vi "Screen.vi"() -> (1 "Screen":bool[][](array[boolean]))   [LabVIEW 2012]
panel:
  # "This screen is 100 x 150"
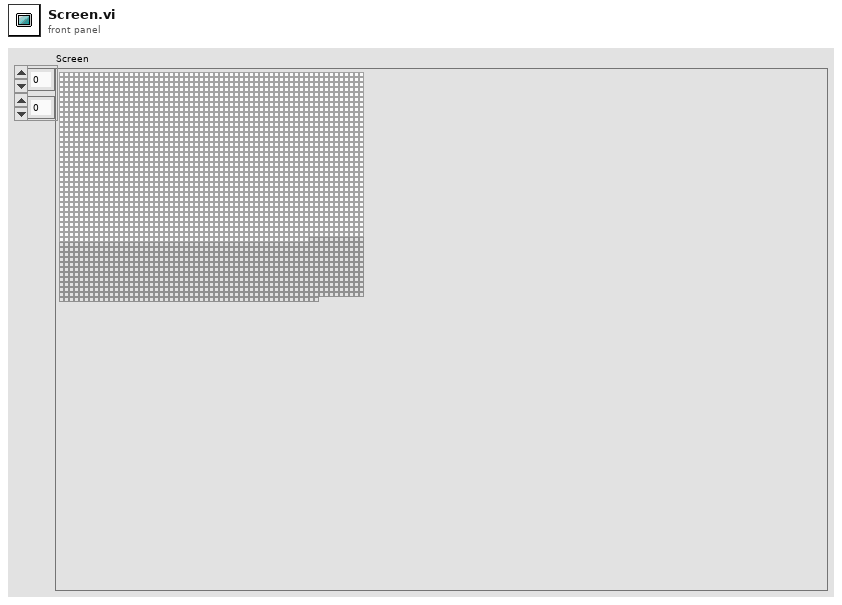
[diagram p1: front panel]
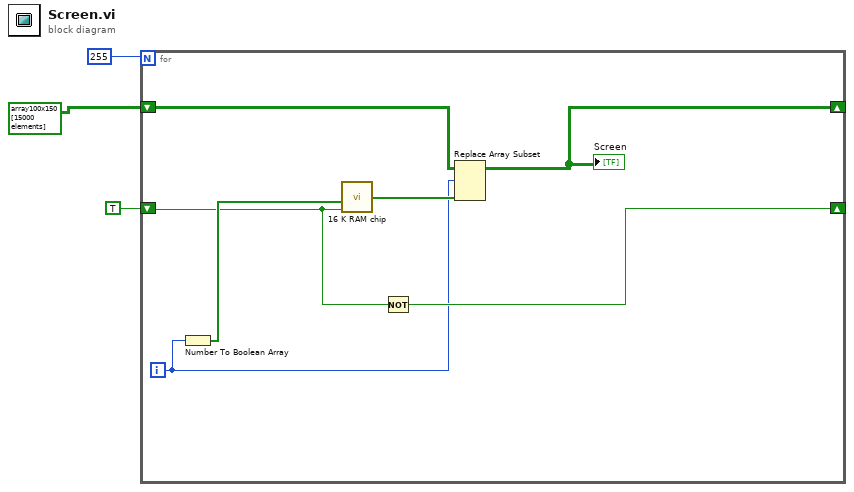
[diagram p0: block diagram]
diagram:
  n1 = for {
    N: u8 255 -> [_]
    shift-right: [w8] -> _
    shift-left: bool[][] array100x150[15000 elements] ("Screen") -> [w9]
    shift-right: [w5] -> _
    shift-left: TRUE -> [w6]
    i -> [w4]
    n2 = Number To Boolean Array(number=w4) -> (Boolean array=w7:bool[])
    n3 = call "16 K RAM chip.vi"("Clock"=w6, "Address"=w7) -> ("Reg Out 1"=w10:bool[])  [unwired: 2 in]
    n4 = Not(x=w6) -> (.not. x?=w5:bool)
    n5 = Replace Array Subset(array=w9, new element=w10, index (row)=w4) -> (w8:bool[][])  [unwired: 1 in]
    "Screen" <- w8
  }
